vi "Read Scale.vi"(9 "Slide in":refnum<class "Slide.lvclass">) -> (3 "Slide out":refnum<class "Slide.lvclass">, 4 "Scale":refnum<class "Scale.lvclass">)   [LabVIEW 2014, in "Slide.lvclass"]
uses:
  Slide.lvclass
  Scale/Scale.lvclass
  Slide.lvclass/Slide.ctl
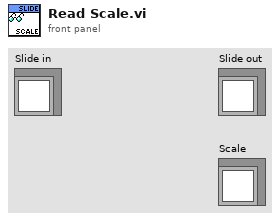
[diagram p1: front panel]
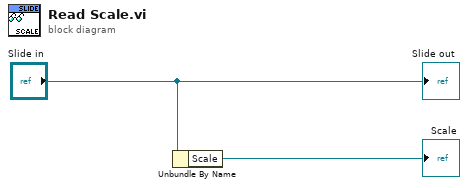
[diagram p0: block diagram]
diagram:
  n1 = Unbundle By Name("Slide in") -> ("Scale"=→"Scale":refnum<class "Scale.lvclass">)
  "Slide out" <- "Slide in"
